vi "Modbus_Shutdown.vi"(0 "MB session in":refnum<class "MB_Master.lvclass">, 3 "error in (no error)":errorcluster) -> (10 "error out":errorcluster)   [LabVIEW 2026]
uses:
  <vilib>/Plasmionique/MB Master/MB_Master/MB_Master.lvclass
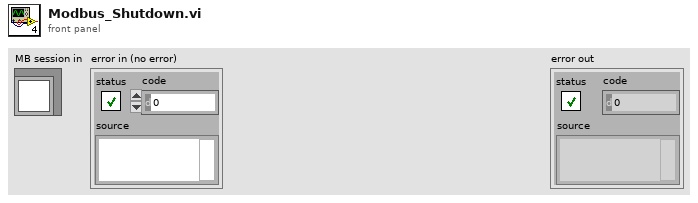
[diagram p1: front panel]
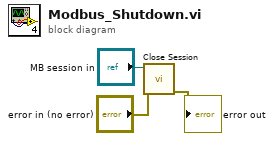
[diagram p0: block diagram]
diagram:
  n1 = call-dynamic "Close Session.vi"("error in (no error)"="error in (no error)", "MB session in"="MB session in") -> ("error out"=→"error out":errorcluster)  [unwired: 9 in]
